vi "toString.vi"(8 "error in (no error)":errorcluster, 11 "iMessage in":refnum<class "iMessage.lvclass">) -> (0 "error out":errorcluster, 2 "String":string, 3 "iMessage out":refnum<class "iMessage.lvclass">)   [LabVIEW 2017, in "Message Interface.lvlib" / "iMessage.lvclass"]
uses:
  iMessage.lvclass
  iMessage.lvclass/iMessage.ctl
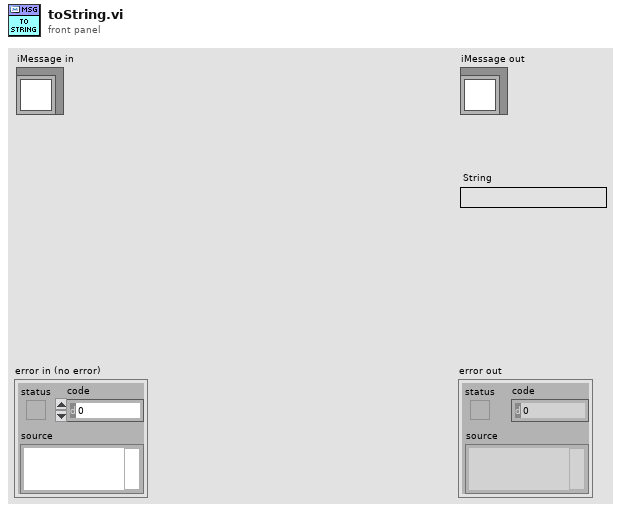
[diagram p1: front panel]
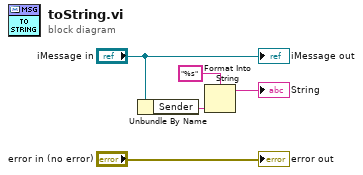
[diagram p0: block diagram]
diagram:
  n1 = Unbundle By Name("iMessage in") -> ("Sender"=w3:string)
  n2 = Format Into String(format string="%s", w3) -> (resulting string=→"String":string)  [unwired: 2 in, 1 out]
  "error out" <- "error in (no error)"
  "iMessage out" <- "iMessage in"
